vi "SBML_Events_Parser.vi"(6 "error in (no error)":errorcluster, 8 "Input SBML File":string) -> (0 "error out":errorcluster, 1 "Event Info":string[][](table), 3 "Event_cnt":i32)   [LabVIEW 2014]
doc: "This VI extract the information of reactions present in SBML file. It takes the complete SBML file as input, and outputs: \nReac_Cnt --> How many reactions are there\nReac_Id_Arr --> Array of reactions\nReac_rev_Arr --> Indicates if the corresponding indexed reaction is reversible\nReac_fast --> Indicates if the corresponding indexed reaction is fast\nKinetic Laws --> Extract the list of kinetic laws of each reaction\nModifiers_Arr --> Array of modifiers (or catalysts)\nProducts_Arr --> Array of products of reactions\n\nDesigned by HB\nhaba@dtu.dk"
panel:
  out "Delay":string[](array[string])
  out "Priority":string[](array[string])
  out "Assignment":string[](array[string])
  out "initialValue ?":string[](array[string])
  out "Order":string[](array[string])
  out "Trigger Math":string[](array[string])
  out "Persistent ?":string[](array[string])
  out "Value From Trigger Time":string[](array[string])
  out "Event_Id_Arr":string[](array[string])
  out "List of Events":string
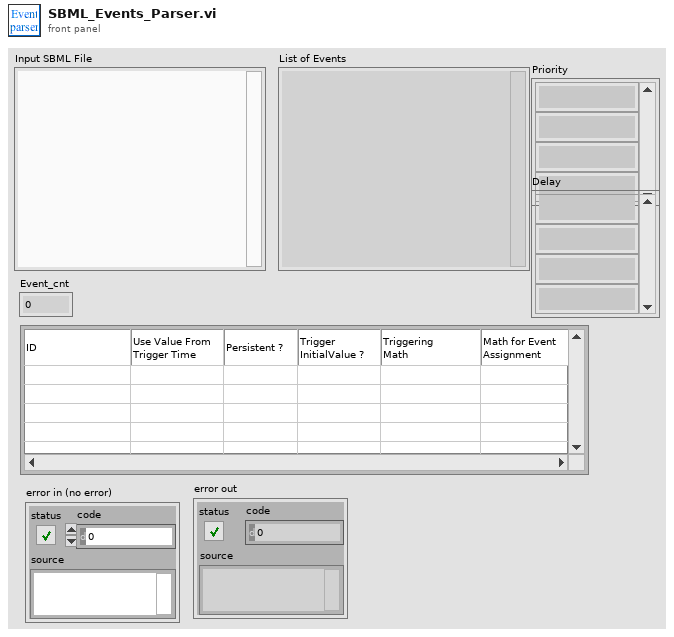
[diagram p1: front panel]
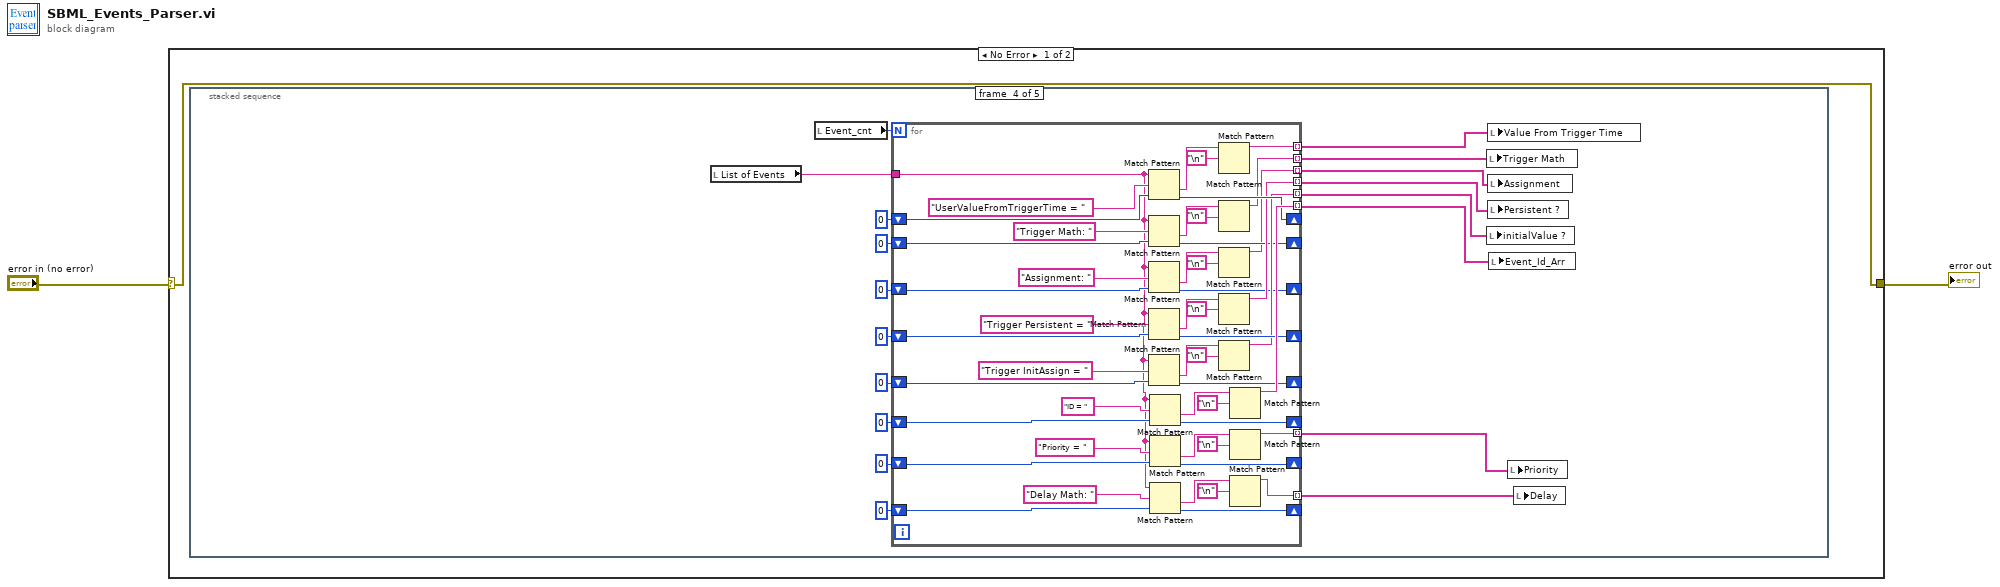
[diagram p0: block diagram]
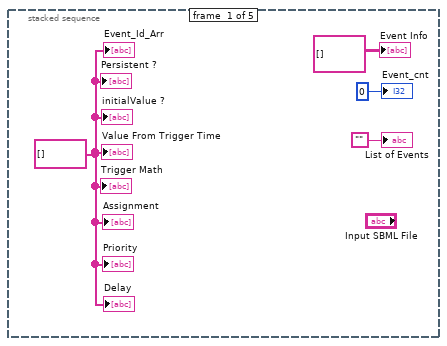
[diagram p2: hidden frame]
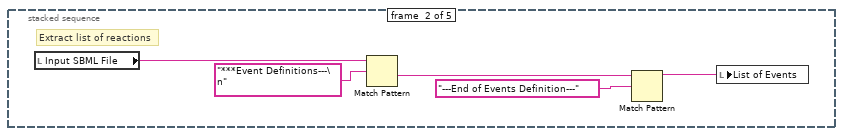
[diagram p3: hidden frame]
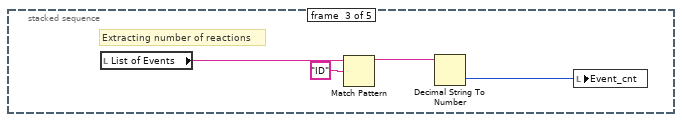
[diagram p4: hidden frame]
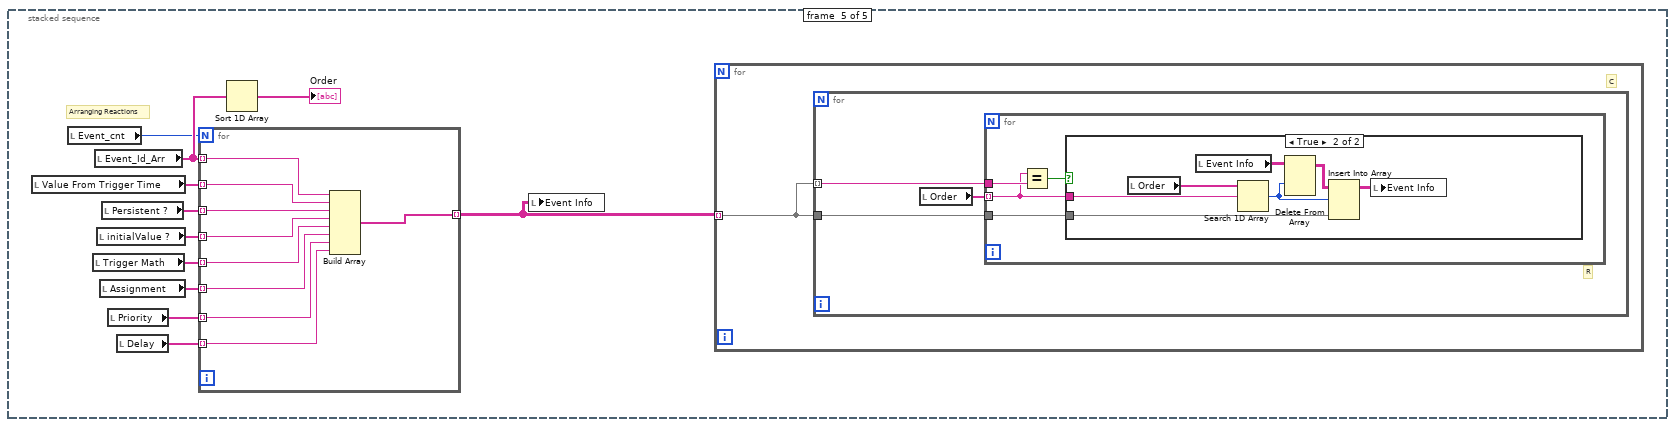
[diagram p5: hidden frame]
diagram:
  n1 = case shown="No Error" "error in (no error)" {
    selector: "error in (no error)" -> [w3 w119]
    tunnel: [w3 w119] -> w1
    frame No Error {
      n2 = stacked-sequence {
        frame #0 {
          w4 = string[] [] ("Sp_Id_Arr")
          "List of Events" <- "" ("Full SBML File")
          "Event_cnt" <- 0 ("Reac_cnt")
          "Event_Id_Arr" <- w4
          "Value From Trigger Time" <- w4
          "Persistent ?" <- w4
          "Trigger Math" <- w4
          "Event Info" <- string[][] [] ("Reaction Info")
          "initialValue ?" <- w4
          "Assignment" <- w4
          "Priority" <- w4
          "Delay" <- w4
        }
        frame #1 {
          # "Extract list of reactions"
          n3 = local read "Input SBML File"() -> (w12:string)
          n4 = Match Pattern(string=w12, regular expression="***Event Definitions---\n") -> (after substring=w10:string)  [unwired: 1 in, 3 out]
          n5 = Match Pattern(string=w10, regular expression="---End of Events Definition---") -> (before substring=w8:string)  [unwired: 1 in, 3 out]
          n6 = local write "List of Events"(w8) -> ()
        }
        frame #2 {
          # "Extracting number of reactions"
          n7 = local read "List of Events"() -> (w14:string)
          n8 = Match Pattern(string=w14, regular expression="ID") -> (before substring=w16:string)  [unwired: 1 in, 3 out]
          n9 = Decimal String To Number(string=w16) -> (number=w13:i32)  [unwired: 2 in, 1 out]
          n10 = local write "Event_cnt"(w13) -> ()
        }
        frame #3 {
          n11 = local read "List of Events"() -> (w34:string)
          n12 = local read "Event_cnt"() -> (w33:i32)
          n13 = for {
            N: w33 -> [_]
            tunnel: w34 -> [w35]
            shift-right: [w79] -> _
            shift-left: 0 ("offset of match") -> [w80]
            tunnel: [w78] -> w31 mode=indexing
            shift-right: [w76] -> _
            shift-left: 0 ("offset of match") -> [w75]
            tunnel: [w77] -> w29 mode=indexing
            shift-right: [w67] -> _
            shift-left: 0 ("offset of match") -> [w68]
            tunnel: [w66] -> w21 mode=indexing
            shift-right: [w64] -> _
            shift-left: 0 ("offset of match") -> [w63]
            tunnel: [w65] -> w24 mode=indexing
            shift-right: [w55] -> _
            shift-left: 0 ("offset of match") -> [w56]
            tunnel: [w54] -> w23 mode=indexing
            shift-right: [w52] -> _
            shift-left: 0 ("offset of match") -> [w51]
            tunnel: [w53] -> w22 mode=indexing
            shift-right: [w47] -> _
            shift-left: 0 ("offset of match") -> [w46]
            shift-right: [w38] -> _
            shift-left: 0 ("offset of match") -> [w39]
            tunnel: [w37] -> w18 mode=indexing
            tunnel: [w36] -> w17 mode=indexing
            n14 = Match Pattern(string=w35, regular expression="UserValueFromTriggerTime = ", offset (0)=w75) -> (after substring=w72:string, offset past match=w76:i32)  [unwired: 2 out]
            n15 = Match Pattern(string=w35, regular expression="Trigger Math: ", offset (0)=w56) -> (after substring=w59:string, offset past match=w55:i32)  [unwired: 2 out]
            n16 = Match Pattern(string=w35, regular expression="Assignment: ", offset (0)=w51) -> (after substring=w48:string, offset past match=w52:i32)  [unwired: 2 out]
            n17 = Match Pattern(string=w35, regular expression="Trigger Persistent = ", offset (0)=w68) -> (after substring=w71:string, offset past match=w67:i32)  [unwired: 2 out]
            n18 = Match Pattern(string=w35, regular expression="Trigger InitAssign = ", offset (0)=w63) -> (after substring=w60:string, offset past match=w64:i32)  [unwired: 2 out]
            n19 = Match Pattern(string=w35, regular expression="ID = ", offset (0)=w80) -> (after substring=w83:string, offset past match=w79:i32)  [unwired: 2 out]
            n20 = Match Pattern(string=w35, regular expression="Priority = ", offset (0)=w46) -> (after substring=w43:string, offset past match=w47:i32)  [unwired: 2 out]
            n21 = Match Pattern(string=w35, regular expression="Delay Math: ", offset (0)=w39) -> (after substring=w42:string, offset past match=w38:i32)  [unwired: 2 out]
            n22 = Match Pattern(string=w72, regular expression="\n") -> (before substring=w77:string)  [unwired: 1 in, 3 out]
            n23 = Match Pattern(string=w59, regular expression="\n") -> (before substring=w54:string)  [unwired: 1 in, 3 out]
            n24 = Match Pattern(string=w48, regular expression="\n") -> (before substring=w53:string)  [unwired: 1 in, 3 out]
            n25 = Match Pattern(string=w71, regular expression="\n") -> (before substring=w66:string)  [unwired: 1 in, 3 out]
            n26 = Match Pattern(string=w60, regular expression="\n") -> (before substring=w65:string)  [unwired: 1 in, 3 out]
            n27 = Match Pattern(string=w83, regular expression="\n") -> (before substring=w78:string)  [unwired: 1 in, 3 out]
            n28 = Match Pattern(string=w43, regular expression="\n") -> (before substring=w37:string)  [unwired: 1 in, 3 out]
            n29 = Match Pattern(string=w42, regular expression="\n") -> (before substring=w36:string)  [unwired: 1 in, 3 out]
          }
          n30 = local write "Trigger Math"(w23) -> ()
          n31 = local write "initialValue ?"(w24) -> ()
          n32 = local write "Value From Trigger Time"(w29) -> ()
          n33 = local write "Assignment"(w22) -> ()
          n34 = local write "Persistent ?"(w21) -> ()
          n35 = local write "Event_Id_Arr"(w31) -> ()
          n36 = local write "Priority"(w18) -> ()
          n37 = local write "Delay"(w17) -> ()
        }
        frame #4 {
          # "Arranging Reactions"
          n38 = local read "Value From Trigger Time"() -> (w90:string[])
          n39 = local read "Event_cnt"() -> (w89:i32)
          n40 = local read "Trigger Math"() -> (w87:string[])
          n41 = local read "Event_Id_Arr"() -> (w93:string[])
          n42 = local read "initialValue ?"() -> (w92:string[])
          n43 = local read "Assignment"() -> (w86:string[])
          n44 = local read "Persistent ?"() -> (w91:string[])
          n45 = local read "Priority"() -> (w85:string[])
          n46 = local read "Delay"() -> (w84:string[])
          n47 = for {
            N: w89 -> [_]
            tunnel: w93 -> [w118] mode=indexing
            tunnel: w90 -> [w117] mode=indexing
            tunnel: w91 -> [w116] mode=indexing
            tunnel: w92 -> [w115] mode=indexing
            tunnel: [w114] -> w88 mode=indexing
            tunnel: w87 -> [w113] mode=indexing
            tunnel: w86 -> [w112] mode=indexing
            tunnel: w85 -> [w111] mode=indexing
            tunnel: w84 -> [w110] mode=indexing
            n48 = Build Array(w118, w117, w116, w115, w113, w112, w111, w110) -> (w114:string[])
          }
          n49 = Sort 1D Array(array=w93) -> (sorted array=→"Order":string[])
          n50 = local write "Event Info"(w88) -> ()
          n51 = for {
            tunnel: w88 -> [w95] mode=indexing
            # "C"
            n52 = for {
              tunnel: w95 -> [w97] mode=indexing
              tunnel: w95 -> [w96]
              # "R"
              n53 = local read "Order"() -> (w98:string[])
              n54 = for {
                tunnel: w98 -> [w100] mode=indexing
                tunnel: w97 -> [w102]
                tunnel: w96 -> [w99]
                n55 = Equal?(x=w100, y=w102) -> (x = y?=w101:bool)
                n56 = case shown="True" w101 {
                  tunnel: w100 -> [_ w108]
                  tunnel: w99 -> [_ w107]
                  frame False {
                  }
                  frame True {
                    n57 = local read "Order"() -> (w109:string[])
                    n58 = local read "Event Info"() -> (w105:string[][])
                    n59 = Search 1D Array(1D array=w109, element=w108) -> (index of element=w104:i32)  [unwired: 1 in]
                    n60 = Delete From Array(array=w105, index (row)=w104) -> (array with subset deleted=w103:string[][])  [unwired: 2 in, 1 out]
                    n61 = Insert Into Array(array=w103, index (row)=w104, new element=w107) -> (w106:string[][])  [unwired: 1 in]
                    n62 = local write "Event Info"(w106) -> ()
                  }
                }
              }
            }
          }
        }
      }
    }
    frame Error {
    }
  }
  "error out" <- w1
